vi "Eliminated.vi"(6 "Column":i32, 8 "Row":i32, 9 "Killer Index":i32, 10 "Team Index":i32, 11 "Square in":refnum<class "Square.lvclass">) -> (3 "Square out":refnum<class "Square.lvclass">)   [LabVIEW 2020, in "Square.lvclass"]
uses:
  Square.lvclass
  Type Defs/Status Enum.ctl
  SubVIs/SB SubVIs.lvlib
  Type Defs/SB Type Defs.lvlib
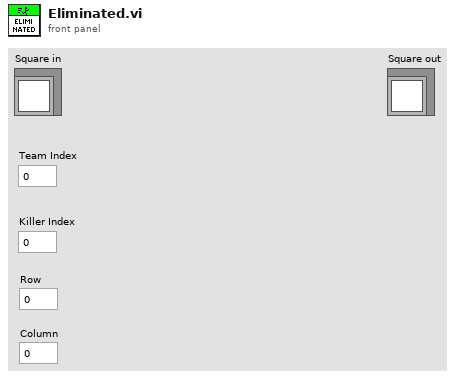
[diagram p1: front panel]
types:
  T1 = typedef "SB Type Defs.lvlib/Status Enum.ctl" = enum16{"Replicate", "Kill", "Eliminate", "Collide"}
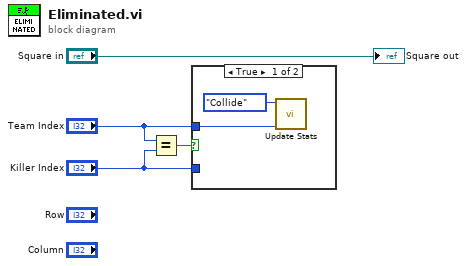
[diagram p0: block diagram]
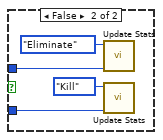
[diagram p2: hidden frame]
diagram:
  n1 = Equal?(x="Team Index", y="Killer Index") -> (x = y?=w4:bool)
  n2 = case shown="True" w4 {
    tunnel: "Team Index" -> [w6 w10]
    tunnel: "Killer Index" -> [_ w7]
    frame True {
      n3 = call "Update Stats.vi"("Team"=w6, "Enum"=Status_Enum."Collide") -> ()  [unwired: 10 in]
    }
    frame False {
      n4 = call "Update Stats.vi"("Team"=w10, "Enum"=Status_Enum."Eliminate") -> ()  [unwired: 10 in]
      n5 = call "Update Stats.vi"("Team"=w7, "Enum"=Status_Enum."Kill") -> ()  [unwired: 10 in]
    }
  }
  "Square out" <- "Square in"
